vi "Read states.vi"(8 "error in (no error)":errorcluster, 11 "PositionTactic in":refnum<class "PositionTactic.lvclass">) -> (0 "error out":errorcluster, 2 "Enum":T1, 3 "PositionTactic out":refnum<class "PositionTactic.lvclass">)   [LabVIEW 2023, in "PositionTactic.lvclass"]
uses:
  PositionTactic.lvclass
  PositionTactic.lvclass/PositionTactic.ctl
  C:/Users/ebert/Documents/codes/SSL/repo/SSL_AI/NewSTP/NewTactics/Tactic_v2_class/Tactic_v2.lvclass
  C:/Users/ebert/Documents/codes/SSL/repo/SSL_AI/PositionTactic_class/PositionTactic.lvclass
  PositionTactic_states/PositionTactic_states.ctl
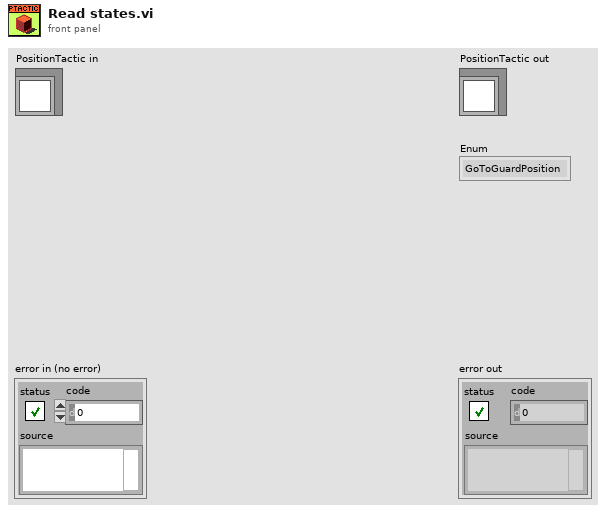
[diagram p1: front panel]
types:
  T1 = typedef "PositionTactic.lvclass/PositionTactic_states.ctl" = enum16{"GoToGuardPosition", "GoToTarget", "Exit"}
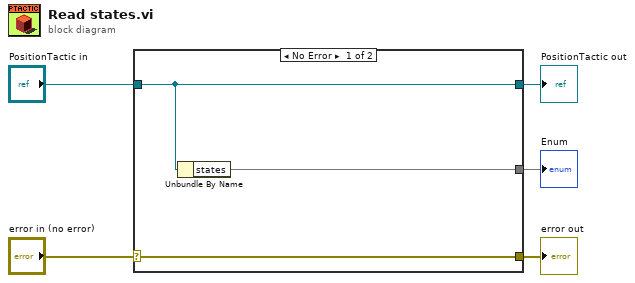
[diagram p0: block diagram]
diagram:
  n1 = case shown="No Error" "error in (no error)" {
    selector: "error in (no error)" -> [w8 w9]
    tunnel: [w8 w9] -> w4
    tunnel: [w7 w10] -> w2
    tunnel: "PositionTactic in" -> [w7 w10]
    tunnel: [w6 _] -> w1
    frame No Error {
      n2 = Unbundle By Name(w7) -> ("states"=w6)
    }
    frame Error {
    }
  }
  "error out" <- w4
  "PositionTactic out" <- w2
  "Enum" <- w1
